vi "Instantiate LV RT.vi"   [LabVIEW 2016, in "Document.lvclass"]
uses:
  Document.lvclass
  Child Classes/LV Doc/Child Classes/LV RT/LV RT.lvclass
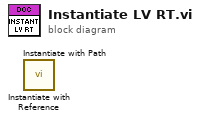
[diagram p0: block diagram]
diagram:
  n1 = call "Instantiate with Reference.vi"() -> ()  [unwired: 14 in, 2 out]
  n2 = call "Instantiate with Path.vi"() -> ()  [unwired: 14 in, 2 out]
